vi "Get Output Enable.vi"(0 "object in":refnum<class "HPS-17000-PowerModule.lvclass">, 11 "Error In":errorcluster) -> (4 "object out":refnum<class "HPS-17000-PowerModule.lvclass">, 6 "output":bool, 15 "Error Out":errorcluster)   [LabVIEW 2023, in "HPS-17000-PowerModule.lvlib" / "HPS-17000-PowerModule.lvclass"]
uses:
  HPS-17000-PowerModule.lvclass
  <instrlib>/HPS-17000/Internal/Get Enabled Output Multi.vi
  <instrlib>/HPS-17000/HPS-17000.lvclass
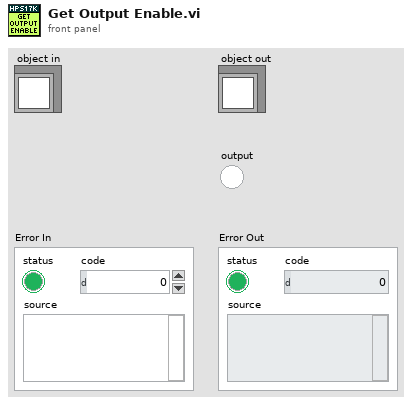
[diagram p1: front panel]
types:
  T1 = typedef "HPS-17000-PowerModule.lvlib/HPS-17000-PowerModule.lvclass/ObjectAttributes.ctl" = cluster{"HPS17000 IP Addresses":string[], "HPS Topology":enum16{"SINGLE", "MULTI"}, "GM ID":string, "TSN NIC IP Address":string, "HPS17000 Refs":refnum<class "HPS-17000.lvclass">[], "Stream Queues":refnum<queue>[], "connected":bool, "reserved":bool, "events":T2, "nibatterycycler_grpc_Setpoint":T3, "last timestamp":i64, "setpoint stream config":T4, "mode":T5, "range":T6}
  T2 = typedef "HPS-17000.lvclass/Multi-Cycler Events.ctl" = cluster{"heartbeats events":refnum<user-event>[], "faults events":refnum<user-event>[], "network sync event":refnum<user-event>[], "setpoint status event":refnum<user-event>[]}
  T3 = typedef "NI_BC_client.lvlib/nibatterycycler_grpc_Setpoint.ctl" = cluster{"voltage":sgl, "current":sgl, "min_power":sgl, "max_power":sgl, "resistance":sgl}
  T4 = typedef "Cycler.lvclass/Setpoint Stream Basic Config.ctl" = cluster{"local address":string, "receiver port":u16}
  T5 = typedef "HPS-17000-PowerModule.lvlib/HPS-17000-PowerModule.lvclass/Mode.ctl" = u16
  T6 = typedef "PowerModuleInterface.lvlibp/PowerModuleInterface.lvclass/Range.ctl" = cluster{"Current Max (A)":dbl, "Current Min (A)":dbl, "Voltage Max (V)":dbl, "Voltage Min (V)":dbl}
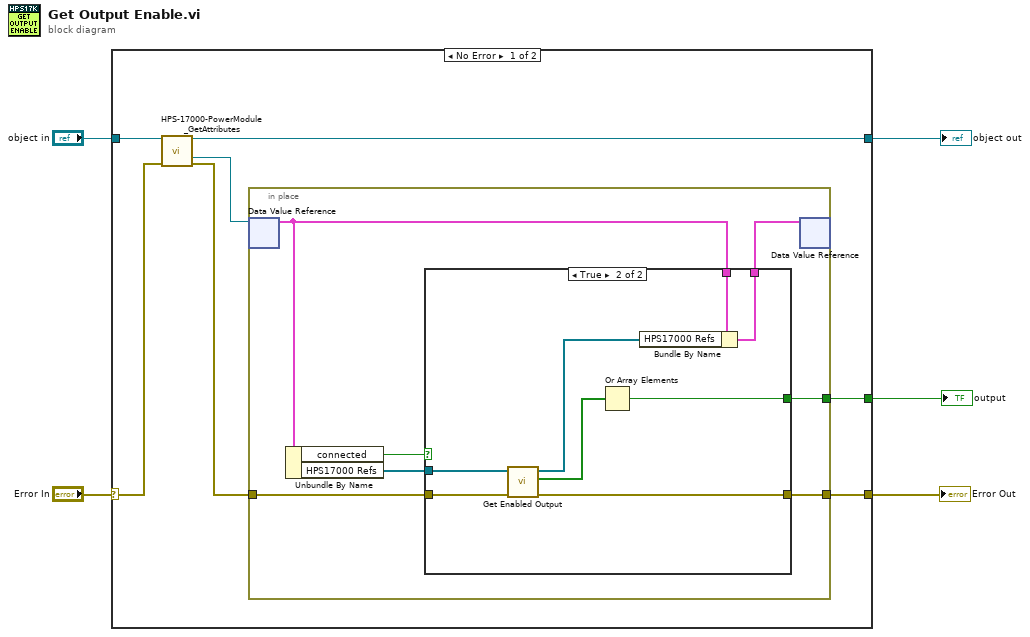
[diagram p0: block diagram]
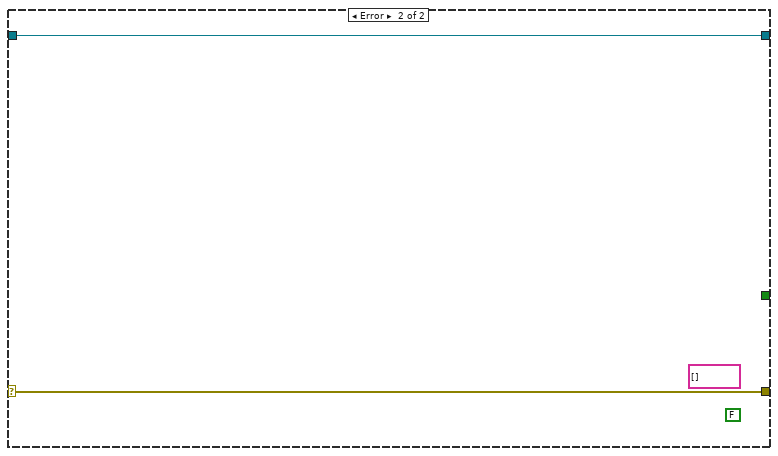
[diagram p3: hidden frame]
diagram:
  n1 = case shown="No Error" "Error In" {
    selector: "Error In" -> [w11 w30]
    tunnel: "object in" -> [w12 w31]
    tunnel: [w7 w31] -> w2
    tunnel: [w8 w30] -> w3
    tunnel: [w6 _] -> w1
    frame No Error {
      n2 = call "HPS-17000-PowerModule_GetAttributes.vi"("reference in"=w12, "Error In"=w11) -> ("reference out"=w7:refnum<class "HPS-17000-PowerModule.lvclass">, "DataRef"=w10:refnum<data-value>, "Error Out"=w9:errorcluster)  [unwired: 10 in, 1 out]
      n3 = in-place {
        in-place-border: w9 -> [w17]
        in-place-border: [w16] -> w8
        in-place-border: [w13] -> w6
        n4 = in-place-dvr #1(w10) -> (w18:T1)  [unwired: 1 out]
        n5 = Unbundle By Name(w18) -> ("connected"=w14:bool, "HPS17000 Refs"=w15:refnum<class "HPS-17000.lvclass">[])
        n6 = case shown="True" w14 {
          tunnel: [w21 w29] -> w19
          tunnel: w18 -> [w21 w28]
          tunnel: w17 -> [w20 w25]
          tunnel: [w20 w22] -> w16
          tunnel: w15 -> [_ w27]
          tunnel: [_ w23] -> w13
          frame False {
          }
          frame True {
            n7 = call-poly <instrlib>:"Get Enabled Output.vi"("error in"=w25, "cycler refs in"=w27) -> ("error out"=w22:errorcluster, "enabled output"=w24:bool[], "cycler refs out"=w26:refnum<class "HPS-17000.lvclass">[])  [unwired: 7 in]
            n8 = Or Array Elements(Boolean array=w24) -> (logical OR=w23:bool)
            n9 = Bundle By Name(cluster=w28, "HPS17000 Refs"=w26) -> (w29:T1)
          }
        }
        n10 = in-place-dvr #1(w19) -> ()  [unwired: 2 out]
      }
    }
    frame Error {
      (unwired) string[] []
      (unwired) FALSE
    }
  }
  "Error Out" <- w3
  "object out" <- w2
  "output" <- w1
